vi "add search path.vi"(8 "error in":errorcluster, 10 "search path":path, 11 "glyph manager in":T1) -> (0 "error out":errorcluster, 3 "glyph manager out":T1)   [LabVIEW 2025, in "CEF.lvlib"]
doc: "Copyright 2017 National Instruments Corporation\n\nLicensed under the Apache License, Version 2.0 (the \"License\"); you may not use this file except in compliance with the License. You may obtain a copy of the License at http://www.apache.org/licenses/LICENSE-2.0\nUnless required by applicable law or agreed to in writing, software distributed under the License is distributed on an \"AS IS\" BASIS, WITHOUT WARRANTIES OR CONDITIONS OF ANY KIND, either express or implied. See the License for the specific language governing permissions and limitations under the License."
uses:
  CEF.lvlib
  glyph manager.ctl
  <vilib>/picture/picture.llb/imagedata.ctl
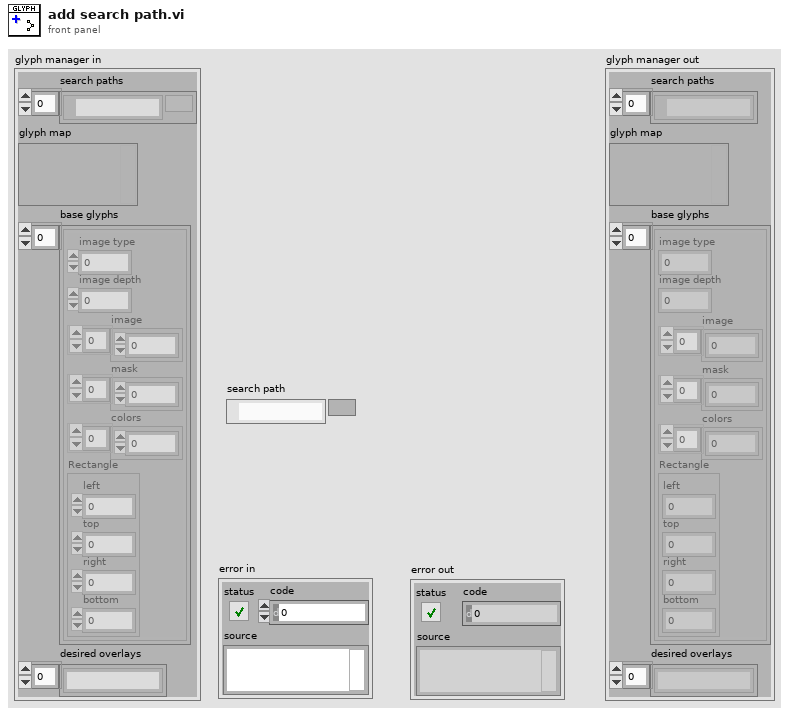
[diagram p1: front panel]
types:
  T1 = typedef "CEF.lvlib/glyph manager.ctl" = cluster{"search paths":path[], "glyph map":variant, "base glyphs":T2[], "desired overlays":string[]}
  T2 = typedef "imagedata.ctl" = cluster{"image type":i32, "image depth":i32, "image":u8[], "mask":u8[], "colors":u32[], "Rectangle":cluster{"left":i16, "top":i16, "right":i16, "bottom":i16}}
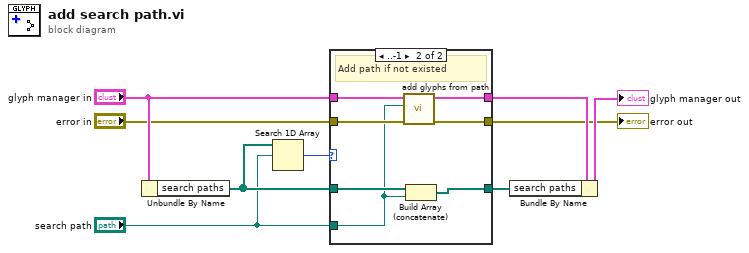
[diagram p0: block diagram]
diagram:
  n1 = Unbundle By Name("glyph manager in") -> ("search paths"=w9:path[])
  n2 = Search 1D Array(1D array=w9, element="search path") -> (index of element=w7:i32)  [unwired: 1 in]
  n3 = case shown="..-1" w7 {
    tunnel: w9 -> [w12 w19]
    tunnel: "search path" -> [_ w13]
    tunnel: [w12 w18] -> w8
    tunnel: "glyph manager in" -> [w10 w17]
    tunnel: [w10 w16] -> w4
    tunnel: "error in" -> [w11 w15]
    tunnel: [w11 w14] -> w1
    frame 0.. {
      # "Do nothing if existed"
    }
    frame ..-1 {
      # "Add path if not existed"
      n4 = call "add glyphs from path.vi"("error in (no error)"=w15, "Path"=w13, "glyph manager in"=w17) -> ("error out"=w14:errorcluster, "glyph manager out"=w16:T1)  [unwired: 7 in]
      n5 = Build Array (concatenate)(w19, w13) -> (w18:path[])
    }
  }
  "error out" <- w1
  n6 = Bundle By Name(cluster=w4, "search paths"=w8) -> (→"glyph manager out":T1)
